vi "New ImageData.vi"(8 "error in (no error)":errorcluster, 10 "ImageData":T1, 11 "CircularBuffer.ImageData":refnum<class "CircularBuffer.ImageData.lvclass">) -> (0 "error out":errorcluster, 2 "newElementIndex":i32=1, 3 "CircularBuffer.ImageData out":refnum<class "CircularBuffer.ImageData.lvclass">)   [LabVIEW 2013, in "CircularBuffer.ImageData.lvclass"]
uses:
  CircularBuffer.ImageData.lvclass
  CircularBuffer/CircularBuffer.lvclass
  <vilib>/picture/picture.llb/imagedata.ctl
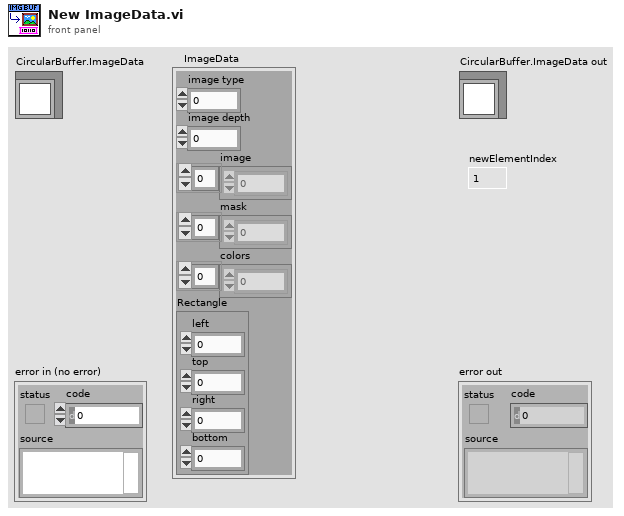
[diagram p1: front panel]
types:
  T1 = typedef "imagedata.ctl" = cluster{"image type":i32, "image depth":i32, "image":u8[], "mask":u8[], "colors":u32[], "Rectangle":cluster{"left":i16, "top":i16, "right":i16, "bottom":i16}}
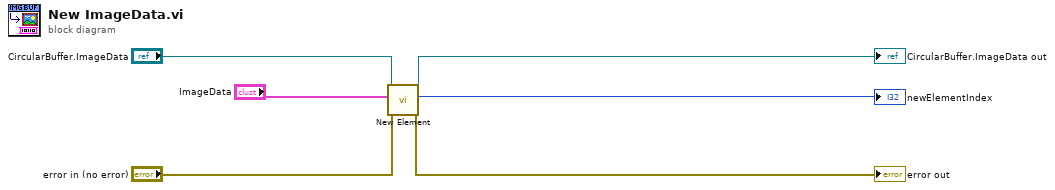
[diagram p0: block diagram]
diagram:
  n1 = call "New Element.vi"("error in (no error)"="error in (no error)", "Element"="ImageData", "CircularBuffer"="CircularBuffer.ImageData") -> ("error out"=→"error out":errorcluster, "newElementIndex"=→"newElementIndex":i32, "CircularBuffer out"=→"CircularBuffer.ImageData out":refnum<class "CircularBuffer.ImageData.lvclass">)  [unwired: 6 in]
